vi "get desired keys.vi"(8 "error in":errorcluster, 11 "GPIC Core configuration in":refnum<class "GPIC Core configuration.lvclass">) -> (0 "error out":errorcluster, 2 "desired keys":string[](array[string]), 3 "GPIC Core configuration out":refnum<class "GPIC Core configuration.lvclass">)   [LabVIEW 2017, in "GPIC Core configuration.lvclass"]
uses:
  GPIC Core configuration.lvclass
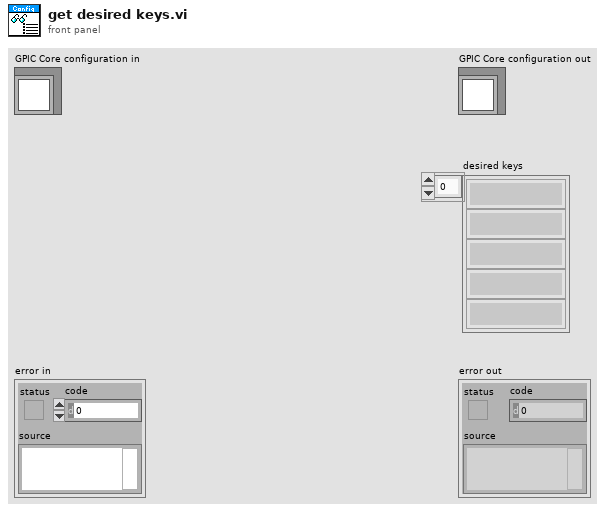
[diagram p1: front panel]
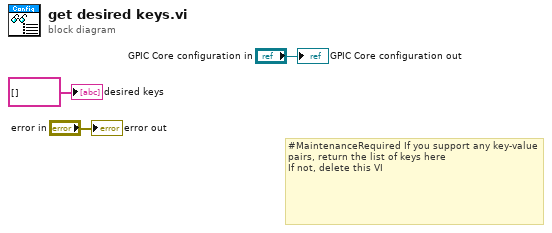
[diagram p0: block diagram]
diagram:
  # "#MaintenanceRequired If you support any key-value pairs, return the list of keys here\nIf not, delete this VI"
  "error out" <- "error in"
  "GPIC Core configuration out" <- "GPIC Core configuration in"
  "desired keys" <- string[] [] ("desired keys")
